vi "RT Main.vi"() -> ()   [LabVIEW 2013]
uses:
  <vilib>/rvi/interface/nirviOpenFPGA/nirviOpenFPGA.xnode
  <vilib>/rvi/interface/nirviReadWriteControl/nirviReadWriteControl.xnode
  <vilib>/myRIO/Instrument Drivers/Utilities/Utilities.lvlib
  <vilib>/rvi/interface/nirviCloseFPGA/nirviCloseFPGA.xnode
  NiFpgaLv.dll
  <vilib>/Utility/error.llb/Error Cluster From Error Code.vi
  <vilib>/rvi/interface/Simulation/niFpgaSimulationCallBeginRW.vi
  <vilib>/rvi/errors/niLvFpgaAdjustHostInterfaceError.vi
  <vilib>/FPGAPlugInAG/Dynamic/niLvFpga_Close_Dynamic.vi
  myRIO with FPGA/myRIO-1900 Customized FPGA.vi
panel:
  in  "Numeric":i64
  out "error out":errorcluster
  out "SYS.RDY":bool
  out "Acceleration":T1(graph)
  in  "Stop Button":bool
  # "Overview: The myRIO Custom FPGA Project template acquires acceleration data from the onboard accelerometer and displays the changes of acceleration values in a waveform chart. The SYS.RDY indicator shows the FPGA status.\nRequirements: LabVIEW FPGA Module.\nInstructions:\n1. Check the myRIO target IP Address in the project and make sure the target IP Address is correct. \n2. Run the VI."
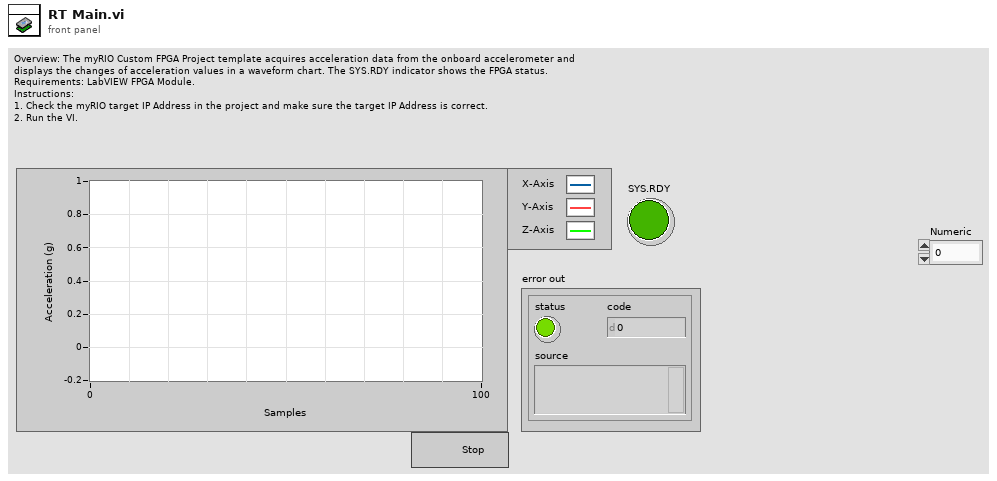
[diagram p1: front panel]
types:
  T1 = cluster{"X-Axis":dbl, "Y-Axis":dbl, "Z-Axis":dbl}
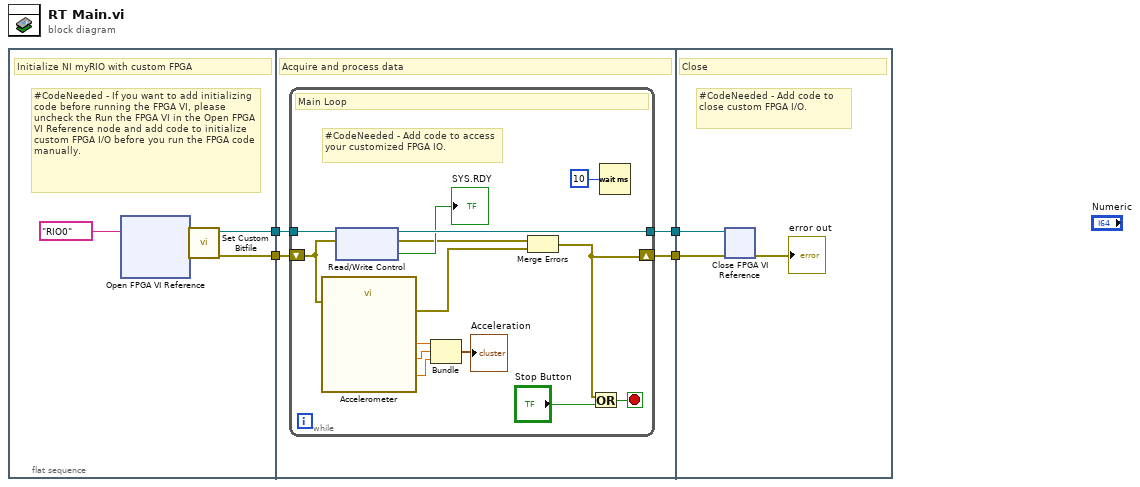
[diagram p0: block diagram]
diagram:
  n1 = flat-sequence {
    tunnel: [w5] -> w4
    tunnel: [w6] -> w3
    tunnel: w4 -> [w13]
    tunnel: w3 -> [w12]
    tunnel: [w11] -> w2
    tunnel: [w10] -> w1
    tunnel: w2 -> [w30]
    tunnel: w1 -> [w29]
    frame #0 {
      # "#CodeNeeded - If you want to add initializing code before running the FPGA VI, please uncheck the Run the FPGA VI in the Open FPGA VI Reference node and add code to initialize custom FPGA I/O before you run the FPGA code manually."
      # "Initialize NI myRIO with custom FPGA"
      n2 = xnode "Open FPGA VI Reference"("resource name"=tag "RIO0") -> ("FPGA VI Reference Out"=w7:refnum<k20>, "error out"=w8:errorcluster)  [unwired: 1 in]
      n3 = call <vilib>:"Set Custom Bitfile.vi"("error in (no error)"=w8, "Customized FPGA Reference in"=w7) -> ("error out"=w5:errorcluster, "Customized FPGA Reference out"=w6:refnum<k20>)  [unwired: 8 in]
    }
    frame #1 {
      # "Acquire and process data"
      n4 = while {
        tunnel: w12 -> [w25]
        tunnel: [w23] -> w11
        shift-right: [w20] -> w10
        shift-left: w13 -> [w14]
        stop <- w26 stop-if-true
        # "#CodeNeeded - Add code to access your customized FPGA IO."
        # "Main Loop"
        n5 = call "Accelerometer"("error in (no error)"=w14) -> ("X-Axis"=w19:dbl, "Y-Axis"=w17:dbl, "Z-Axis"=w18:dbl, "error out"=w15:errorcluster)  [unwired: 23 in]
        n6 = xnode "Read/Write Control"("FPGA VI Reference In"=w25, "error in"=w14) -> ("FPGA VI Reference Out"=w23:refnum<k20>, "error out"=w21:errorcluster, "SYS.RDY"=→"SYS.RDY":bool)
        n7 = Bundle("X-Axis"=w19, "Y-Axis"=w17, "Z-Axis"=w18) -> (→"Acceleration":T1)  [unwired: 1 in]
        n8 = Merge Errors(w21, w15) -> (w20:errorcluster)
        n9 = Or(x=w20, y="Stop Button") -> (x .or. y?=w26:bool)
        n10 = Wait (ms)(milliseconds to wait=u32 10) -> ()  [unwired: 1 out]
      }
    }
    frame #2 {
      # "#CodeNeeded - Add code to close custom FPGA I/O."
      # "Close"
      n11 = xnode "Close FPGA VI Reference"("FPGA VI Reference In"=w30, "error in"=w29) -> ("error out"=→"error out":errorcluster)
    }
  }
